vi "Error Query.vi"(8 "error in (no error)":errorcluster, 11 "VISA resource name":refnum<visa-resource-name>) -> (0 "error out":errorcluster, 1 "Error Message":string, 2 "Error Code":i32[](array[numeric]), 3 "VISA resource name out":refnum<visa-resource-name>)   [LabVIEW 2021, in "DmmPwr Simulator.lvlib"]
doc: "Queries the instrument for any errors in the instrument's error queue. It will continue to read errors until all errors have been read from the instrument. Any errors will be returned in the <B>error out</B> control.\n\n<B>Note:</B>\nThis VI is called automatically by most driver VIs so it is not usually necessary to call this in an application."
uses:
  DmmPwr Simulator.lvlib
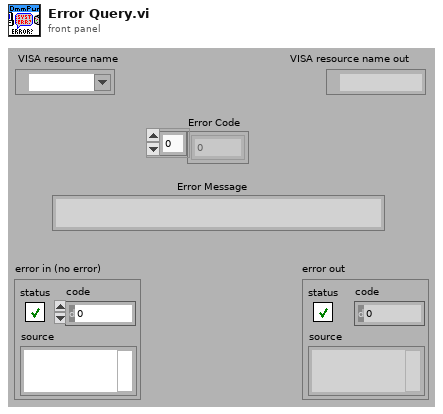
[diagram p1: front panel]
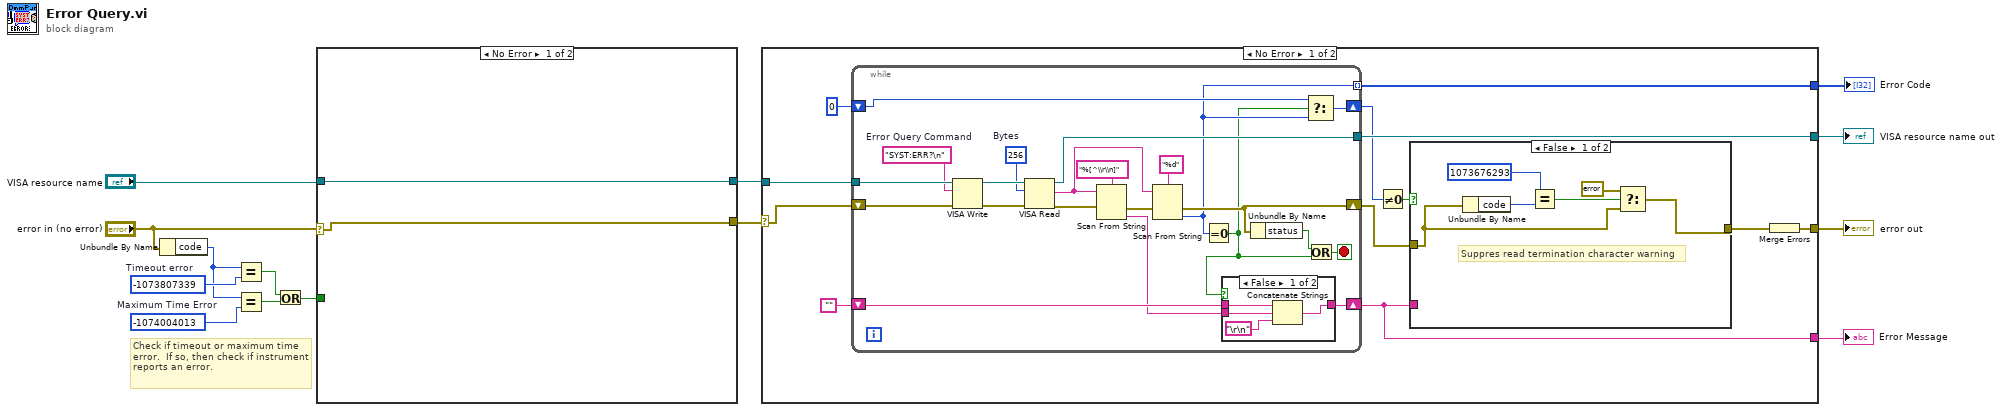
[diagram p0: block diagram]
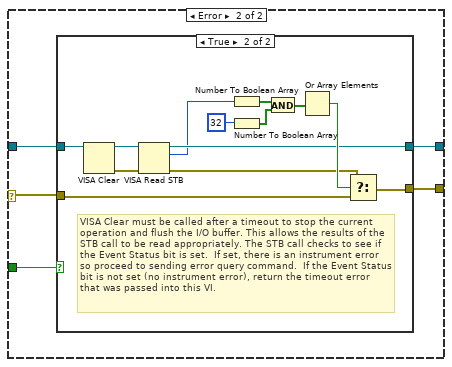
[diagram p2: hidden frame]
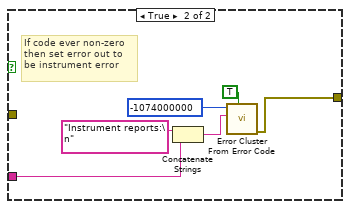
[diagram p4: hidden frame]
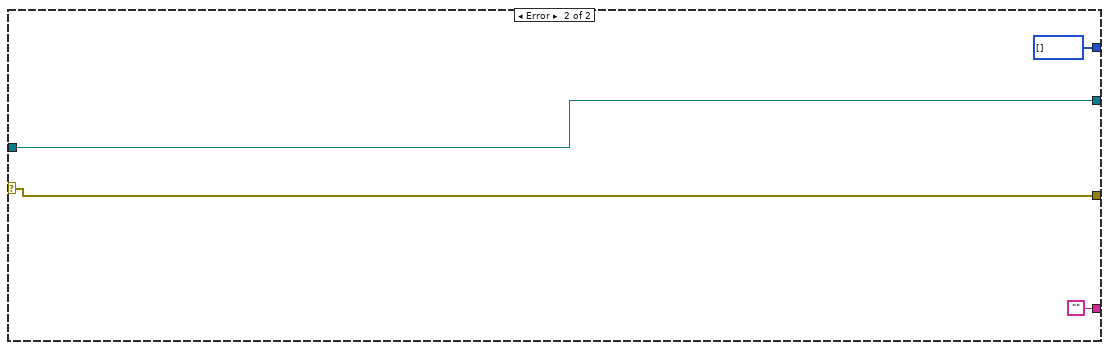
[diagram p6: hidden frame]
diagram:
  w5 = -1074004013  # Maximum Time Error
  w7 = -1073807339  # Timeout error
  # "Check if timeout or maximum time error.  If so, then check if instrument reports an error."
  n1 = Unbundle By Name("error in (no error)") -> ("code"=w6:i32)
  n2 = Equal?(x=w6, y=w7) -> (x = y?=w3:bool)
  n3 = Equal?(x=w6, y=w5) -> (x = y?=w4:bool)
  n4 = Or(x=w3, y=w4) -> (x .or. y?=w2:bool)
  n5 = case shown="No Error" "error in (no error)" {
    selector: "error in (no error)" -> [w15 w19]
    tunnel: "VISA resource name" -> [w16 w21]
    tunnel: [w16 w20] -> w9
    tunnel: [w15 w18] -> w10
    tunnel: w2 -> [_ w17]
    frame No Error {
    }
    frame Error {
      n6 = case shown="True" w17 {
        tunnel: w21 -> [w23 w29]
        tunnel: [w23 w26] -> w20
        tunnel: w19 -> [w22 w32]
        tunnel: [w22 w31] -> w18
        frame False {
          # "Error code not a timeout, so best to pass on to user."
        }
        frame True {
          # "VISA Clear must be called after a timeout to stop the current operation and flush the I/O buffer. This allows the results of the  STB call to be read appropriately. The STB call checks to see if the Event Status bit is set.  If set, there is an instrument error so proceed to sending error query command.  If the Event Status bit is not set (no instrument error), return the timeout error that was passed into this VI."
          n7 = VISA Clear(VISA resource name=w29) -> (VISA resource name out=w28:refnum<visa-resource-name>, error out=w27:errorcluster)  [unwired: 1 in]
          n8 = VISA Read STB(8:w27, 11:w28) -> (0:w25:errorcluster, 2:w24:u16, 3:w26:refnum<visa-resource-name>)
          n9 = Number To Boolean Array(number=w24) -> (Boolean array=w33:bool[])
          n10 = Number To Boolean Array(number=32) -> (Boolean array=w35:bool[])
          n11 = And(x=w33, y=w35) -> (x .and. y?=w34:bool[])
          n12 = Or Array Elements(Boolean array=w34) -> (logical OR=w30:bool)
          n13 = Select(t=w25, s=w30, f=w32) -> (s? t:f=w31:errorcluster)
        }
      }
    }
  }
  n14 = case shown="No Error" w10 {
    selector: w10 -> [w37 w88]
    tunnel: [w48 w91] -> w14
    tunnel: w9 -> [w47 w91]
    tunnel: [w45 w88] -> w13
    tunnel: [w40 ""] -> w12
    tunnel: [w39 i32[] []] -> w11
    frame No Error {
      n15 = while {
        tunnel: [w82] -> w48
        tunnel: w47 -> [w81]
        shift-right: [w70] -> w40
        shift-left: "" -> [w72]
        shift-right: [w68] -> w41
        shift-left: 0 -> [w69]
        shift-right: [w66] -> w38
        shift-left: w37 -> [w67]
        tunnel: [w62] -> w39 mode=indexing
        stop <- w75 stop-if-true
        w79 = u32 256  # Bytes
        w77 = "SYST:ERR?\n"  # Error Query Command
        n16 = VISA Write(VISA resource name=w81, write buffer=w77, error in (no error)=w67) -> (VISA resource name out=w80:refnum<visa-resource-name>, error out=w78:errorcluster)  [unwired: 1 out]
        n17 = VISA Read(VISA resource name=w80, byte count=w79, error in (no error)=w78) -> (VISA resource name out=w82:refnum<visa-resource-name>, read buffer=w73:string, error out=w65:errorcluster)  [unwired: 1 out]
        n18 = Scan From String(format string="%[^\\r\\n]", input string=w73, error in=w65) -> (error out=w64:errorcluster, output 1=w71:string)  [unwired: 2 in, 2 out]
        n19 = Scan From String(format string="%d", input string=w73, error in=w64) -> (error out=w66:errorcluster, output 1=w62:i32)  [unwired: 2 in, 2 out]
        n20 = Equal To 0?(x=w62) -> (x = 0?=w61:bool)
        n21 = case shown="False" w61 {
          tunnel: w72 -> [w86 w87]
          tunnel: w71 -> [w84 _]
          tunnel: [w83 w87] -> w70
          frame False {
            n22 = Concatenate Strings(w86, w84, "\r\n") -> (w83:string)
          }
          frame True {
          }
        }
        n23 = Unbundle By Name(w66) -> ("status"=w63:bool)
        n24 = Select(t=w69, s=w61, f=w62) -> (s? t:f=w68:i32)
        n25 = Or(x=w63, y=w61) -> (x .or. y?=w75:bool)
      }
      n26 = Not Equal To 0?(x=w41) -> (x != 0?=w43:bool)
      n27 = case shown="False" w43 {
        tunnel: w40 -> [_ w59]
        tunnel: [w49 w55] -> w42
        tunnel: w38 -> [w51 _]
        frame False {
          # "Suppres read termination character warning"
          n28 = Unbundle By Name(w51) -> ("code"=w54:i32)
          n29 = Equal?(x=1073676293, y=w54) -> (x = y?=w52:bool)
          n30 = Select(t=errorcluster {"status"=FALSE, "code"=0, "source"=""}, s=w52, f=w51) -> (s? t:f=w49:errorcluster)
        }
        frame True {
          # "If code ever non-zero\nthen set error out to\nbe instrument error"
          n31 = Concatenate Strings("Instrument reports:\n" ("Source"), w59) -> (w56:string)
          n32 = call <vilib>:"Error Cluster From Error Code.vi"("show call chain? (False)"=TRUE, "error message (\"\")"=w56, "error code (0)"=-1074000000 ("Code")) -> ("error out"=w55:errorcluster)  [unwired: 6 in]
        }
      }
      n33 = Merge Errors(w42) -> (w45:errorcluster)
    }
    frame Error {
    }
  }
  "VISA resource name out" <- w14
  "error out" <- w13
  "Error Message" <- w12
  "Error Code" <- w11
